vi "Read ADU Packet.vi"(8 "error in (no error)":errorcluster, 10 "protocol layer":refnum<class "Network Protocol.lvclass">, 11 "IP transmission data unit in":refnum<class "IP Data Unit.lvclass">) -> (0 "error out":errorcluster, 1 "modbus data unit":refnum<class "Modbus Data Unit (PDU).lvclass">, 2 "protocol layer out":refnum<class "Network Protocol.lvclass">, 3 "IP transmission data unit out":refnum<class "IP Data Unit.lvclass">, 5 "PDU Valid?":bool)   [LabVIEW 2020, in "SubVIs.lvlib" / "IP Data Unit.lvclass"]
doc: "This uses the protocol layer to read a modbus packet off of the bus, wrapped in the IP transmission data unit."
uses:
  <vilib>/Modbus/subvis/Transmission Data Unit (ADU)/IP Data Unit/IP Data Unit.lvclass
  C:/builds/penguin/iak/lvdsc/trunk/20.0/lv/vi.lib/Modbus/subvis/Transmission Data Unit (ADU)/Transmission Data Unit/Transmission Data Unit.lvclass
  <vilib>/Modbus/subvis/Modbus Data Unit (PDU)/Modbus Data Unit (PDU).lvclass
  <vilib>/Modbus/subvis/Protocol/Interfaces/Network Protocol/Network Protocol.lvclass
  <vilib>/Modbus/subvis/Transmission Data Unit (ADU)/Transmission Data Unit/Transmission Data Unit.lvclass/Transmission Data Unit.ctl
  <vilib>/Modbus/subvis/Transmission Data Unit (ADU)/IP Data Unit/IP Data Unit.lvclass/IP Data Unit.ctl
  <vilib>/Modbus/subvis/Modbus Data Unit (PDU)/Modbus Data Unit (PDU).lvclass/Modbus Data Unit (PDU).ctl
  <vilib>/Utility/error.llb/Error Cluster From Error Code.vi
  <vilib>/ErrorRing/Error Ring.xnode
  <vilib>/Modbus/subvis/Transmission Data Unit (ADU)/Transmission Data Unit/Transmission Data Unit.lvclass
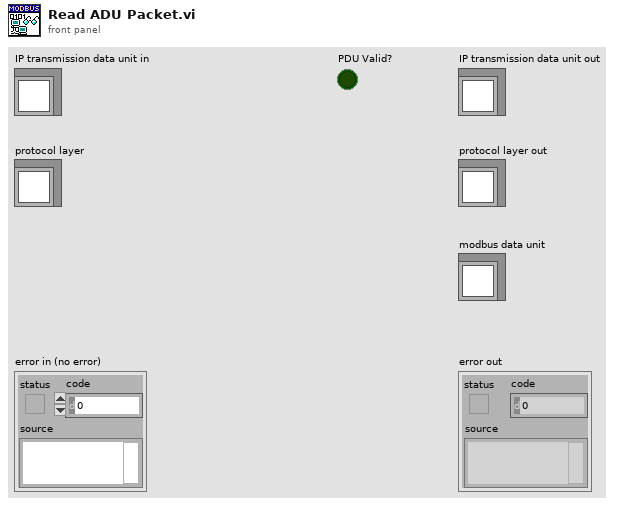
[diagram p1: front panel]
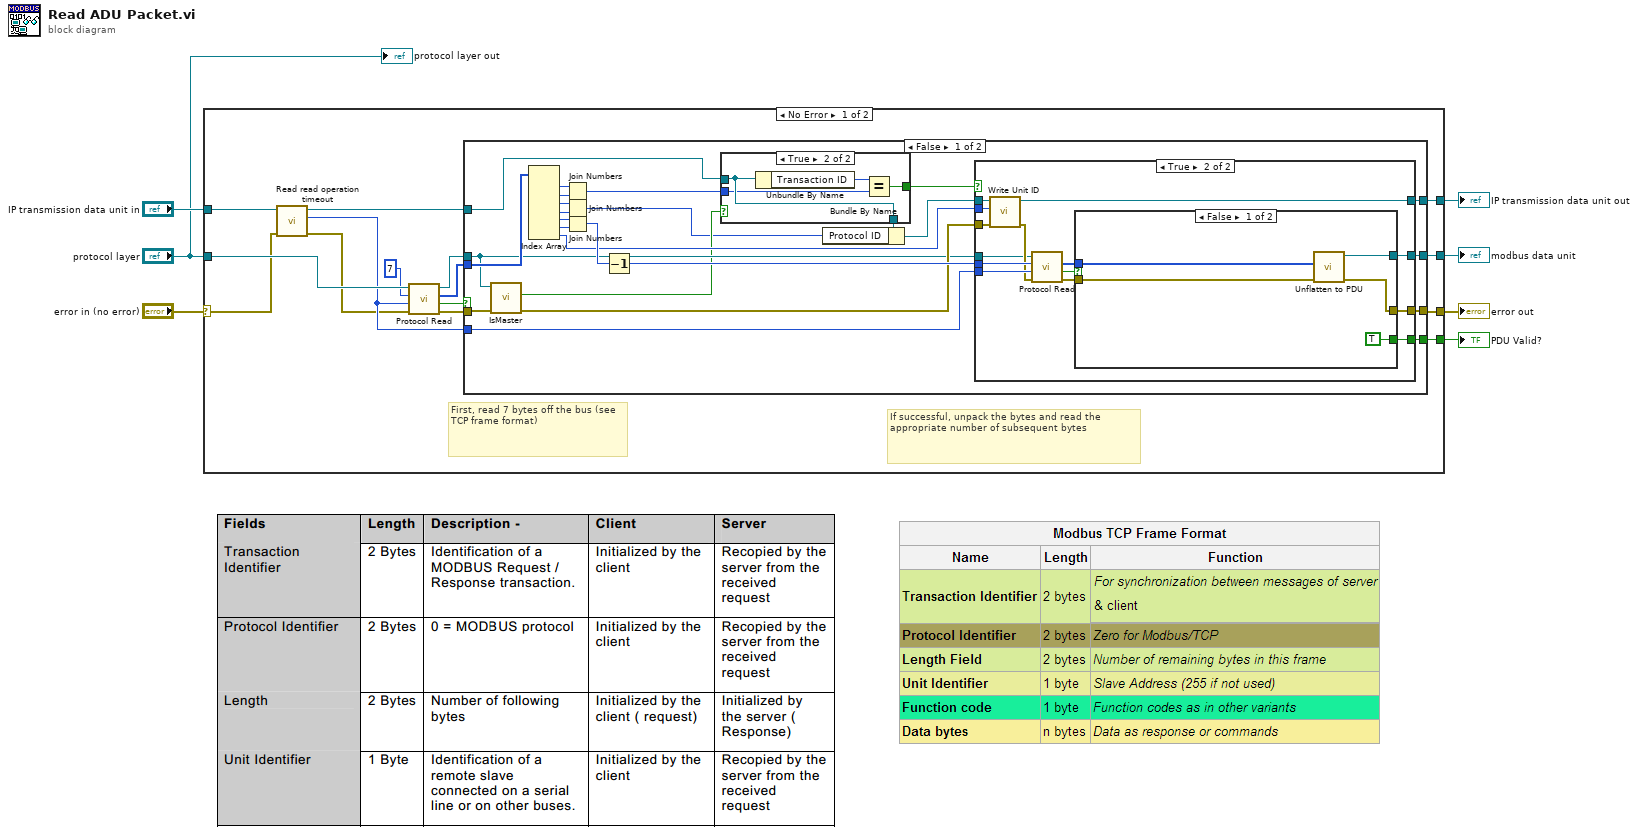
[diagram p0: block diagram]
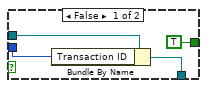
[diagram p2: hidden frame]
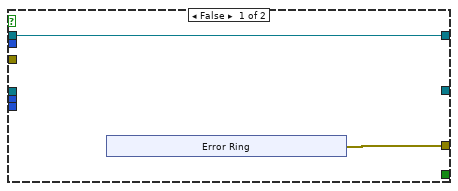
[diagram p3: hidden frame]
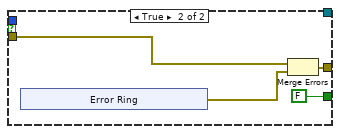
[diagram p4: hidden frame]
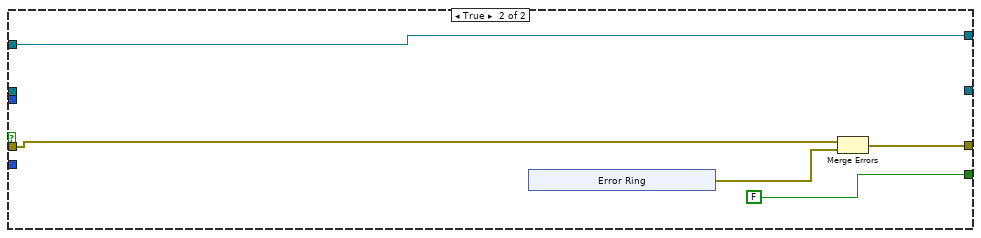
[diagram p5: hidden frame]
diagram:
  n1 = case shown="No Error" "error in (no error)" {
    selector: "error in (no error)" -> [w10 w99]
    tunnel: [w16 w99] -> w6
    tunnel: "IP transmission data unit in" -> [w12 w98]
    tunnel: [w19 w98] -> w4
    tunnel: "protocol layer" -> [w22 _]
    tunnel: [w15 _] -> w3
    tunnel: [w8 _] -> w1
    frame No Error {
      # "If successful, unpack the bytes and read the appropriate number of subsequent bytes"
      # "First, read 7 bytes off the bus (see TCP frame format)"
      n2 = call <vilib>:"Read read operation timeout.vi"("error in (no error)"=w10, "transmission data unit in"=w12) -> ("error out"=w9:errorcluster, "read operation timeout"=w13:i32, "transmission data unit out"=w11:refnum<class "IP Data Unit.lvclass">)  [unwired: 7 in]
      n3 = call-dynamic "Protocol Read.vi"("error in (no error)"=w9, "timeout"=w13, "bytes to read"=7 ("Bytes to Read"), "protocol layer in"=w22) -> ("error out"=w17:errorcluster, "timed out?"=w14:bool, "data"=w20:u8[], "protocol layer out"=w18:refnum<class "Network Protocol.lvclass">)  [unwired: 4 in]
      n4 = case shown="False" w14 {
        tunnel: w20 -> [w47 _]
        tunnel: w11 -> [w26 w93]
        tunnel: [w35 w93] -> w19
        tunnel: w18 -> [w30 _]
        tunnel: w13 -> [w39 _]
        tunnel: w17 -> [w32 w90]
        tunnel: [w37 w91] -> w16
        tunnel: [w36 _] -> w15
        tunnel: [w33 FALSE] -> w8
        frame False {
          n5 = call-dynamic "IsMaster.vi"("error in (no error)"=w32, "Network Protocol in"=w30) -> ("error out"=w31:errorcluster, "isMaster"=w29:bool)  [unwired: 7 in, 1 out]
          n6 = Index Array(array=w47) -> (element #1=w45:u8, element #2=w46:u8, element #3=w44:u8, element #4=w43:u8, element #5=w41:u8, element #6=w42:u8, element #7=w34:u8)  [unwired: 7 in]
          n7 = Join Numbers(hi=w45, lo=w46) -> ((hi.lo)=w28:u16)
          n8 = Join Numbers(hi=w44, lo=w43) -> ((hi.lo)=w25:u16)
          n9 = Join Numbers(hi=w41, lo=w42) -> ((hi.lo)=w40:u16)
          n10 = Decrement(x=w40) -> (x-1=w38:u16)
          n11 = case shown="True" w29 {
            tunnel: w26 -> [w51 w54]
            tunnel: w28 -> [w50 w52]
            tunnel: [TRUE w55] -> w27
            tunnel: [w48 w54] -> w23
            frame False {
              n12 = Bundle By Name(cluster=w51, "Transaction ID"=w50) -> (w48:refnum<class "IP Data Unit.lvclass">)
            }
            frame True {
              n13 = Unbundle By Name(w54) -> ("Transaction ID"=w53:u16)
              n14 = Equal?(x=w53, y=w52) -> (x = y?=w55:bool)
            }
          }
          n15 = Bundle By Name(cluster=w23, "Protocol ID"=w25) -> (w24:refnum<class "IP Data Unit.lvclass">)
          n16 = case shown="True" w27 {
            tunnel: w39 -> [_ w75]
            tunnel: w38 -> [_ w74]
            tunnel: [w56 w72] -> w37
            tunnel: [_ w71] -> w36
            tunnel: w24 -> [w57 w68]
            tunnel: [w57 w67] -> w35
            tunnel: w34 -> [_ w65]
            tunnel: [_ w64] -> w33
            tunnel: w31 -> [_ w63]
            tunnel: w30 -> [_ w62]
            frame False {
              n17 = xnode "Error Ring"() -> ("error out"=w56:errorcluster)
            }
            frame True {
              n18 = call <vilib>:"Write Unit ID.vi"("error in (no error)"=w63, "unit ID"=w65, "transmission data unit in"=w68) -> ("error out"=w66:errorcluster, "transmission data unit out"=w67:refnum<class "IP Data Unit.lvclass">)  [unwired: 7 in]
              n19 = call-dynamic "Protocol Read.vi"("error in (no error)"=w66, "timeout"=w75, "bytes to read"=w74, "protocol layer in"=w62) -> ("error out"=w73:errorcluster, "timed out?"=w69:bool, "data"=w70:u8[])  [unwired: 4 in, 1 out]
              n20 = case shown="False" w69 {
                tunnel: w73 -> [w80 w83]
                tunnel: [w79 w84] -> w72
                tunnel: [w78 _] -> w71
                tunnel: w70 -> [w77 _]
                tunnel: [TRUE FALSE] -> w64
                frame False {
                  n21 = call <vilib>:"Unflatten to PDU.vi"("error in (no error)"=w80, "Modbus data unit data"=w77) -> ("error out"=w79:errorcluster, "Modbus data unit out"=w78:refnum<class "Modbus Data Unit (PDU).lvclass">)  [unwired: 8 in]
                }
                frame True {
                  n22 = xnode "Error Ring"() -> ("error out"=w82:errorcluster)
                  n23 = Merge Errors(w83, w82) -> (w84:errorcluster)
                }
              }
            }
          }
        }
        frame True {
          n24 = xnode "Error Ring"() -> ("error out"=w92:errorcluster)
          n25 = Merge Errors(w90, w92) -> (w91:errorcluster)
        }
      }
    }
    frame Error {
    }
  }
  "error out" <- w6
  "IP transmission data unit out" <- w4
  "modbus data unit" <- w3
  "PDU Valid?" <- w1
  "protocol layer out" <- "protocol layer"
